vi "ProdaNG.Preference.Set.vi"(8 "error in":errorcluster, 9 "value":i32, 10 "key":string, 11 "dbHandleIn":i32) -> (0 "error out":errorcluster, 3 "dbHandle":i32)   [LabVIEW 2016]
doc: "This function serves for identifying a system, if for example, the name and the Wabco Number of the tested part, or the process id and the sequential number in a process are known. \nParameter:\nhandle is an Integer, which is returned by the function Login() at the creation of a new connection.\nsystemName is the name of the system, as it is deposited in the database. If unknown, NULL must be passed.\nwabcoNumber is a known Wabco number in the database. If unknown, NULL must be passed.\nprocessSequence is the sequential Number in the process. If unknown, 0 must be passed.\nprocessId is the according process id. If unknown, 0 must be passed.\n\nmyIdent is a pointer on an identification structure, if the returncode is 0. The structure must be defined in the calling program. The function tries to identify the system definitely under the aid of the passed parameter, in order to return the resulting id's in MyIdent.\n\nThe function tries to identify the system from the following combinations of the parameter:\nsystemName, \nprocessId, \nsystemName and wabcoNumber, \nprocessId and processSequence \nor from all 4 parameter.\nThe more parameters are set, the bigger is the chance, that the system can be identified.\nReturncodes:\n0 No error\n< 0 ORACLE Error Code\n6 (ERROR_INVALID_HANDLE) in case of an invalid handle\n232 (ERROR_NO_DATA) in case that the system cannot be identified definitely."
uses:
  prodllNG.dll
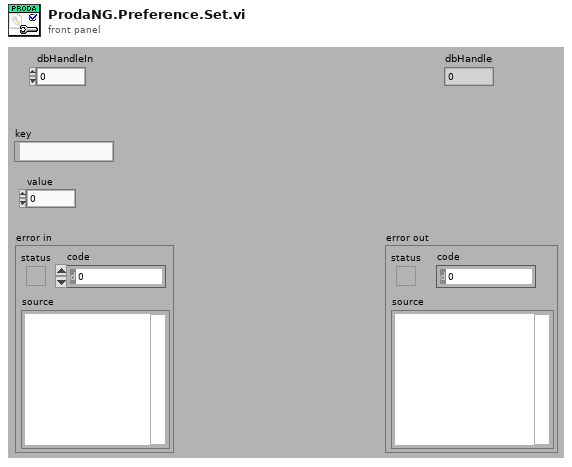
[diagram p1: front panel]
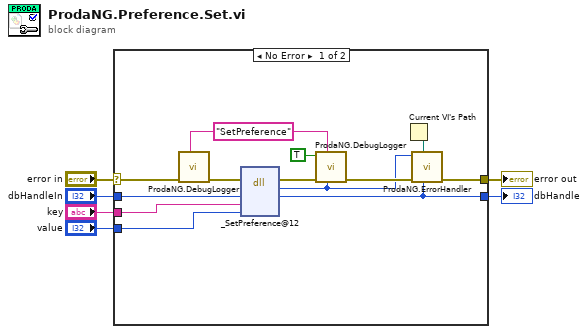
[diagram p0: block diagram]
diagram:
  n1 = case shown="No Error" "error in" {
    selector: "error in" -> [w15 w21]
    tunnel: [w19 w21] -> w5
    tunnel: [w10 w20] -> w4
    tunnel: "dbHandleIn" -> [w9 w20]
    tunnel: "key" -> [w8 _]
    tunnel: "value" -> [w7 _]
    frame No Error {
      w17 = "SetPreference" ("cmd")
      n2 = call "ProdaNG.DebugLogger.vi"("cmd"=w17, "error in (no error)"=w15) -> ("error out"=w14:errorcluster)  [unwired: 9 in]
      n3 = dll-call lib="D:/Maszup/WABCO/SVN/LineTraceSystem/SOFTWARE/sources/Database/ProdaNG/prodllNG.dll" fn="_SetPreference@12" ("ProDll.dll:Login")(error in=w14, "dbHandle"=w9, "key"=w8, "value"=w7) -> (error out=w13:errorcluster, "return type"=w11:i32, "dbHandle"=w10:i32)  [unwired: 4 in, 1 out]
      n4 = call "ProdaNG.DebugLogger.vi"("return type"=w11, "cmd"=w17, "error in (no error)"=w13, "done? (F)"=TRUE) -> ("error out"=w12:errorcluster)  [unwired: 7 in]
      n5 = Current VI's Path() -> (path=w18:path)
      n6 = call "ProdaNG.ErrorHandler.vi"("dbHandleIn"=w10, "Path"=w18, "error in"=w12, "output_parameter"=w11) -> ("error out"=w19:errorcluster)  [unwired: 7 in]
    }
    frame Error {
    }
  }
  "error out" <- w5
  "dbHandle" <- w4
